vi "Create.vi"(8 "error in (no error)":errorcluster, 10 "transfer configuration":T1={"core"={"name"="Transfer"}, "component settings"=[], "channels"=[]} {"channels"."core"."string offset" format="%d bytes"}, 11 "Transfer Configuration in":refnum<class "Transfer Configuration.lvclass">) -> (0 "error out":errorcluster, 3 "Transfer Configuration out":refnum<class "Transfer Configuration.lvclass">)   [LabVIEW 2017, in "DSF Core.lvlib" / "Transfer Configuration.lvclass"]
uses:
  Transfer Configuration.lvclass
  C:/Git/DSF/Core/Classes/Configuration/Core/Core Configuration.lvclass
  Typedefs/DSF Engine Transfer Configuration.ctl
  Typedefs/Core Transfer Configuration.ctl
  Typedefs/DSF Settings Info.ctl
  Typedefs/DSF Engine Channel Configuration.ctl
  Typedefs/Core Channel Configuration.ctl
  Typedefs/DSF Data Type.ctl
  Core Configuration.lvclass/Core Configuration.ctl
  Channel Configuration.ctl
  Transfer Configuration.lvclass/Transfer Configuration.ctl
  Core Configuration.lvclass
  DSF Core.lvlib
  Channel/Channel Configuration.lvclass
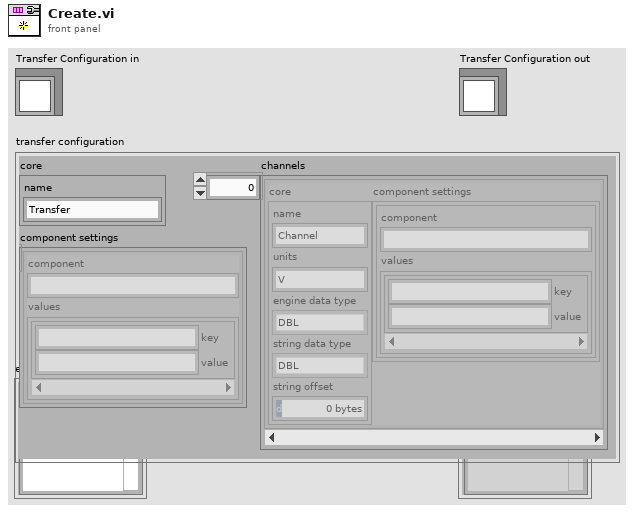
[diagram p1: front panel]
types:
  T1 = typedef "DSF Core.lvlib/DSF Engine Transfer Configuration.ctl" = cluster{"core":T2, "component settings":T3[], "channels":T4[]}
  T2 = typedef "DSF Core.lvlib/Transfer Configuration.lvclass/Core Transfer Configuration.ctl" = cluster{"name":string}
  T3 = typedef "DSF Core.lvlib/DSF Settings Info.ctl" = cluster{"component":string, "values":cluster{"key":string, "value":string}[]}
  T4 = typedef "DSF Core.lvlib/DSF Engine Channel Configuration.ctl" = cluster{"core":T5, "component settings":T3[]}
  T5 = typedef "DSF Core.lvlib/Channel Configuration.lvclass/Core Channel Configuration.ctl" = cluster{"name":string, "units":string, "engine data type":T6, "string data type":T6, "string offset":u64}
  T6 = typedef "DSF Core.lvlib/DSF Data Type.ctl" = enum8{"Bool", "SGL", "DBL", "I8", "I16", "I32", "I64", "U8", "U16", "U32", "U64"}
  T7 = typedef "DSF Core.lvlib/Transfer Configuration.lvclass/Channel Configuration.ctl" = cluster{"configuration":T5, "component settings":T3[]}
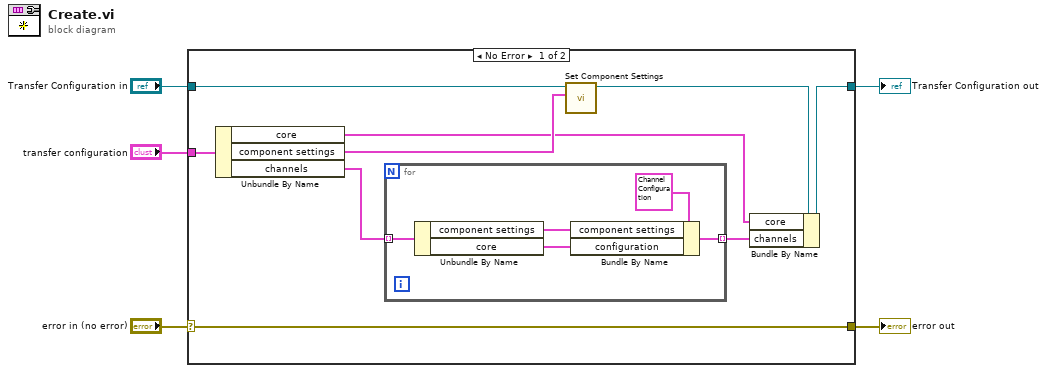
[diagram p0: block diagram]
diagram:
  n1 = case shown="No Error" "error in (no error)" {
    selector: "error in (no error)" -> [w14 w21]
    tunnel: [w14 w21] -> w4
    tunnel: [w13 w20] -> w2
    tunnel: "Transfer Configuration in" -> [w9 w20]
    tunnel: "transfer configuration" -> [w12 _]
    frame No Error {
      n2 = Unbundle By Name(w12) -> ("core"=w6:T2, "component settings"=w10:T3[], "channels"=w8:T4[])
      n3 = for {
        tunnel: w8 -> [w19] mode=indexing
        tunnel: [w17] -> w7 mode=indexing
        n4 = Unbundle By Name(w19) -> ("component settings"=w16:T3[], "core"=w15:T5)
        n5 = Bundle By Name(cluster=T7 {"configuration"={"name"="Channel", "units"="V", "engine data type"=enum."DBL", "string data type"=enum."DBL", "string offset"=0}, "component settings"=[]} ("channel"), "component settings"=w16, "configuration"=w15) -> (w17:T7)
      }
      n6 = call "Set Component Settings.vi"("component settings"=w10, "Runtime Configuration in"=w9) -> ("Runtime Configuration out"=w11:refnum<class "Transfer Configuration.lvclass">)  [unwired: 8 in, 1 out]
      n7 = Bundle By Name(cluster=w11, "core"=w6, "channels"=w7) -> (w13:refnum<class "Transfer Configuration.lvclass">)
    }
    frame Error {
    }
  }
  "error out" <- w4
  "Transfer Configuration out" <- w2
